vi "optionsAcq_interferogramSmoothing.vi"(0 "reference":refnum<class "OSA300.lvclass">, 2 "smoothing":T1, 4 "readWrite":enum16{"read", "write"}(ring), 5 "error in (no error)":errorcluster, 6 "width":u16, 7 "ignore range violation (false)":bool, 8 "nrOfPasses":u16) -> (10 "nrOfPasses out":u16, 12 "width out":u16, 14 "duplicate reference":refnum<class "OSA300.lvclass">, 15 "status":string, 16 "smoothing out":T1, 19 "error out":errorcluster)   [LabVIEW 2010, in "OSA300.lvclass"]
uses:
  OSA300.lvclass
  _misc/Thorlabs_FTS_misc.llb/interferogram_smoothing.ctl
  OSA300.lvclass/OSA300.ctl
  _OSAchannel_class/OSAchannel.lvclass
  OSA.lvclass
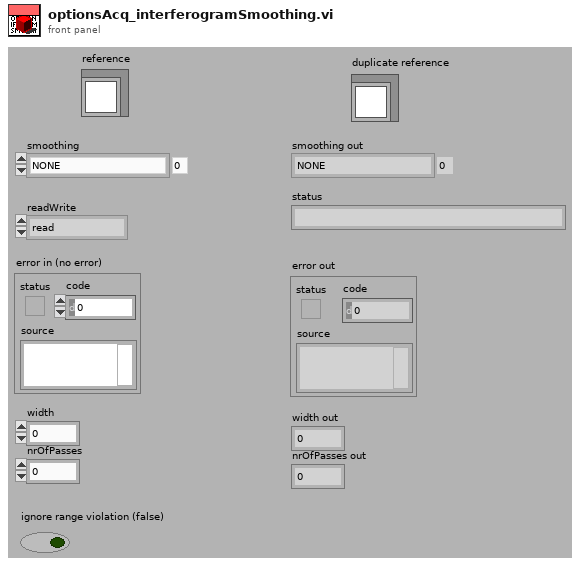
[diagram p1: front panel]
types:
  T1 = typedef "OSA.lvclass/interferogram_smoothing.ctl" = enum16{"NONE", "BINOMIAL", "SAVITSKY_GOLAY", "FOURIER", "MOVING_AVERAGE", "GAUSSIAN"}
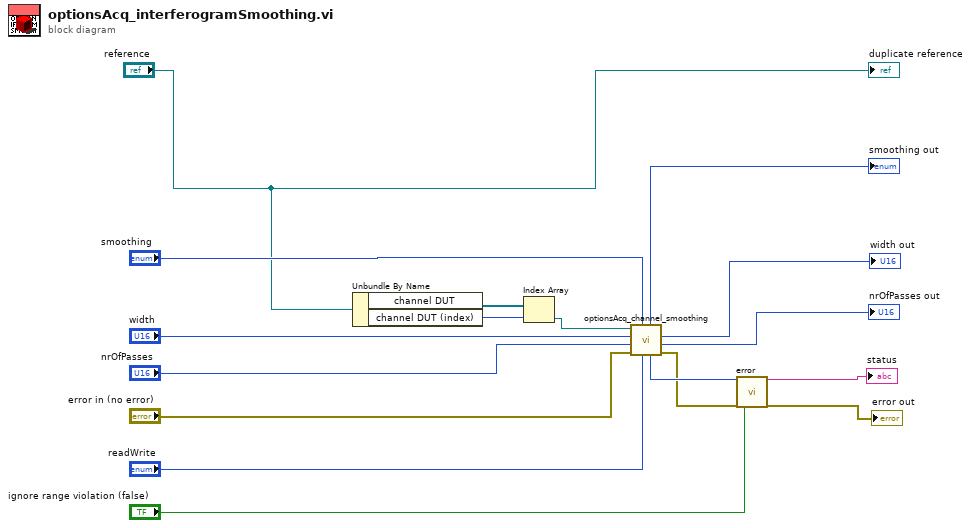
[diagram p0: block diagram]
diagram:
  n1 = Unbundle By Name("reference") -> ("channel DUT"=w17:refnum<class "OSAchannel.lvclass">[], "channel DUT (index)"=w16:i32)
  n2 = Index Array(array=w17, index=w16) -> (element=w15:refnum<class "OSAchannel.lvclass">)
  n3 = call "optionsAcq_channel_smoothing.vi"("readWrite"="readWrite", "smoothing"="smoothing", "error in (no error)"="error in (no error)", "nrOfPasses"="nrOfPasses", "width"="width", "OSAchannel in"=w15) -> ("error out"=w13:errorcluster, "nrOfPasses read"=→"nrOfPasses out":u16, "width read"=→"width out":u16, "FTSLib status"=w14:i32, "smoothing read"=→"smoothing out":T1)  [unwired: 1 out]
  n4 = call "error.vi"("result code"=w14, "error in (no error)"=w13, "ignore range violation"="ignore range violation (false)") -> ("status"=→"status":string, "error out"=→"error out":errorcluster)  [unwired: 14 in, 1 out]
  "duplicate reference" <- "reference"
